vi "Write configuration.vi"(8 "error in":errorcluster, 10 "configuration":refnum<class "NISE_CEF_serializable configuration.lvclass">, 11 "Simple Sequencer TBM editor node in":refnum<class "Simple Sequencer TBM editor node.lvclass">) -> (0 "error out":errorcluster, 3 "Simple Sequencer TBM editor node out":refnum<class "Simple Sequencer TBM editor node.lvclass">)   [LabVIEW 2014, in "Simple Sequencer TBM editor node.lvclass"]
uses:
  Simple Sequencer TBM editor node.lvclass
  <vilib>/NI/Configuration Framework/serializable configuration/NISE_CEF_serializable configuration.lvclass
  module/configuration/Simple Sequencer TBM configuration.lvclass
  Simple Sequencer TBM editor node.lvclass/Simple Sequencer TBM editor node.ctl
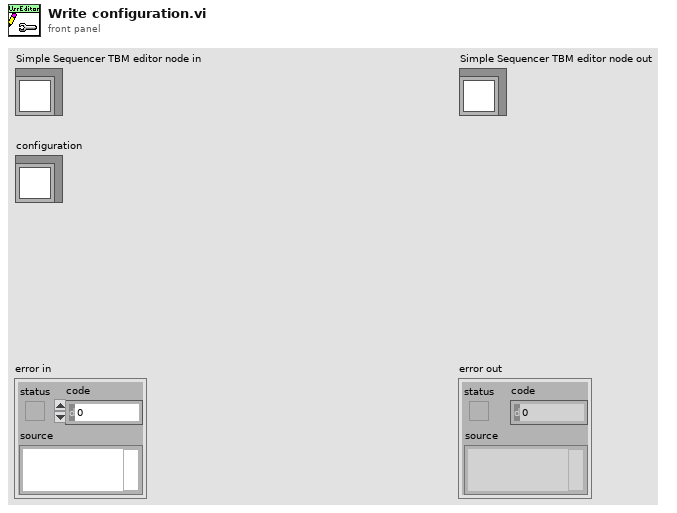
[diagram p1: front panel]
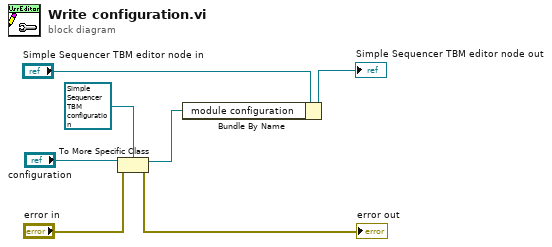
[diagram p0: block diagram]
diagram:
  n1 = To More Specific Class(target class=refnum<class "Simple Sequencer TBM configuration.lvclass"> refnum ("module configuration"), reference="configuration", error in="error in") -> (specific class reference=w3:refnum<class "Simple Sequencer TBM configuration.lvclass">, error out=→"error out":errorcluster)
  n2 = Bundle By Name(cluster="Simple Sequencer TBM editor node in", "module configuration"=w3) -> (→"Simple Sequencer TBM editor node out":refnum<class "Simple Sequencer TBM editor node.lvclass">)
